vi "Output Item Change Event.vi"() -> (3 "Output Value Change Event":refnum<user-event>)   [LabVIEW 2015, in "OutputUI.lvclass"]
uses:
  OutputUI.lvclass
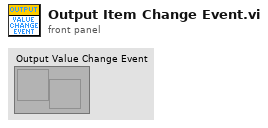
[diagram p1: front panel]
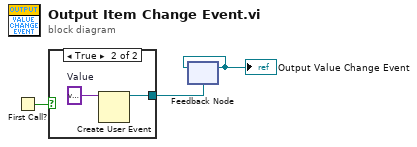
[diagram p0: block diagram]
diagram:
  n1 = First Call?() -> (First Call?: T/F=w2:bool)
  n2 = case shown="True" w2 {
    tunnel: [_ w5] -> w3
    frame False {
    }
    frame True {
      w4 = variant  # Value
      n3 = Create User Event(user event datatype=w4) -> (user event=w5:refnum<user-event>)  [unwired: 1 in, 1 out]
    }
  }
  n4 = feedback #1(w3) -> (w1:refnum<user-event>)
  "Output Value Change Event" <- w1
  n5 = feedback-in #1(w1) -> ()
